vi "GetCurrent.vi"(4 "error in":errorcluster, 5 "connection ID":refnum<k5>) -> (0 "Current":string, 1 "error out":errorcluster, 2 "connection ID out":refnum<k5>, 3 "Answer":bool)   [LabVIEW 2013]
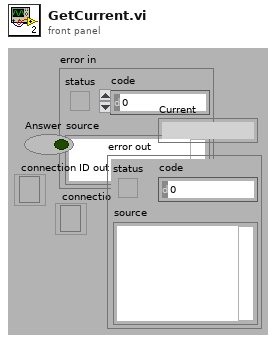
[diagram p1: front panel]
types:
  T1 = enum16{"Standard", "Buffered", "CRLF", "Immediate"}
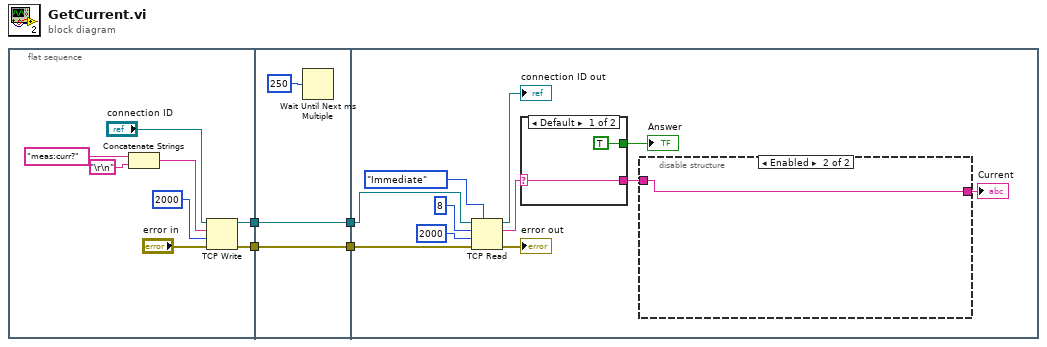
[diagram p0: block diagram]
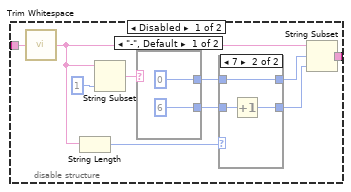
[diagram p2: hidden frame]
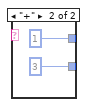
[diagram p4: hidden frame]
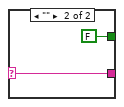
[diagram p5: hidden frame]
diagram:
  n1 = flat-sequence {
    tunnel: [w9] -> w3
    tunnel: [w8] -> w1
    tunnel: [w14] -> w4
    tunnel: w3 -> [w14]
    tunnel: [w13] -> w2
    tunnel: w1 -> [w13]
    tunnel: w4 -> [w19]
    tunnel: w2 -> [w18]
    frame #0 {
      n2 = Concatenate Strings("meas:curr?" ("data in"), "\r\n") -> (w6:string)
      n3 = TCP Write(connection ID="connection ID", data in=w6, error in (no error)="error in", 9:2000 ("timeout ms (25000)")) -> (connection ID out=w9:refnum<k5>, error out=w8:errorcluster)  [unwired: 1 out]
    }
    frame #1 {
      n4 = Wait Until Next ms Multiple(millisecond multiple=u32 250) -> ()  [unwired: 1 out]
    }
    frame #2 {
      n5 = TCP Read(connection ID=w19, bytes to read=8, error in (no error)=w18, 7:T1."Immediate" ("mode (standard)"), 9:2000 ("timeout ms (25000)")) -> (connection ID out=→"connection ID out":refnum<k5>, data out=w24:string, error out=→"error out":errorcluster)
      n6 = case shown="Default" w24 {
        selector: w24 -> [w48 w50]
        tunnel: [w48 w50] -> w17
        tunnel: [TRUE FALSE] -> w23
        frame Default {
        }
        frame "" {
        }
      }
      "Answer" <- w23
      n7 = disable-structure shown="Enabled" {
        disable-tunnel: w17 -> [w28 w46]
        disable-tunnel: [w27 w46] -> w16
        frame Disabled {
          n8 = call <vilib>:"Trim Whitespace.vi"("string"=w28) -> ("trimmed string"=w31:string)  [unwired: 1 in]
          n9 = String Length(string=w31) -> (length=w32:i32)
          n10 = String Subset(string=w31, length (rest)=1 ("length (rest)")) -> (substring=w29:string)  [unwired: 1 in]
          n11 = case shown="\"-\", Default" w29 {
            tunnel: [0 ("length (rest)") 1 ("length (rest)")] -> w35
            tunnel: [6 ("length (rest)") 3 ("length (rest)")] -> w33
            frame "-", Default {
            }
            frame "+" {
            }
          }
          n12 = case shown="7" w32 {
            tunnel: w33 -> [w38 w41]
            tunnel: [w38 w40] -> w34
            tunnel: w35 -> [w37 w39]
            tunnel: [w37 w39] -> w36
            frame 6, Default {
            }
            frame 7 {
              n13 = Increment(x=w41) -> (x+1=w40:i32)
            }
          }
          n14 = String Subset(string=w31, offset (0)=w36, length (rest)=w34) -> (substring=w27:string)
        }
        frame Enabled {
        }
      }
      "Current" <- w16
    }
  }
